vi "GOLPI Package Assistant Panel.vi"(8 "error in":errorcluster, 11 "golpi ref":T1) -> (0 "error out":errorcluster)   [LabVIEW 2013]
doc: "GOLPI package assistant panel."
uses:
  golpi_session_ref.ctl
  golpi_session.ctl
  GOLPI Library.lvlibp/Public/GOLPI reference Type Def.ctl
  GOLPI Library.lvlibp/LV Process source distribution/Pipe Handle.ctl
  GOLPI Library.lvlibp/Private/Get Variable - polymorph parts/Get Double.vi
  <vilib>/regexp/Match Regular Expression.xnode
  GOLPI Multi Process.lvlib
  GOLPI Library.lvlibp
  varilib/varilib.lvlib
  GOLPI Library.lvlibp/LV Process source distribution/LV Process library.lvlib
panel:
  in  "btn install":bool
  in  "btn clr":bool
  in  "btn rem":bool
  in  "btn add":bool
  in  "btn reload":bool
  in  "pkg select":i32(listbox) caption="Packages to load"
  in  "pkg list":i32(listbox) caption="Installed packages"
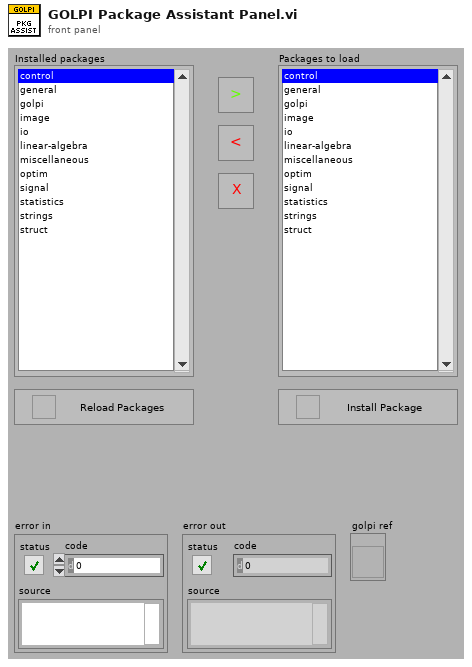
[diagram p1: front panel]
types:
  T1 = typedef "GOLPI Multi Process.lvlib/golpi_session_ref.ctl" = refnum<vi>
  T2 = typedef "GOLPI Package Assistant Actions" = enum16{"Reload packages"}
  T3 = typedef "GOLPI Library.lvlibp/GOLPI reference Type Def.ctl" = cluster{"pipe handle":T4, "fast read timeout [ms]":u32, "fast read settle time [ms]":u32, "fast read to multiple [ms]":u32, "max elements per input line":u32, "slow read timeout [ms]":u32, "stdin double format specifier":string, "max elements per stdout output column":u32, "console mode bitstream":bool, "bitstream first read timeout [ms]":u32, "bitstream read timeout [ms]":u32, "struct transfer possible":bool, "matlab mode":bool}
  T4 = typedef "GOLPI Library.lvlibp/LV Process library.lvlib/Pipe Handle.ctl" = cluster{"lv_proc.dll file path":path, "process instance handle":u32[], "debug mode":bool, "debug data":cluster{"time":timestamp, "stdin":bool, "data":string}[]}
  T5 = typedef "GOLPI Multi Process.lvlib/golpi_session.ctl" = cluster{"GOLPI ref":T3, "idn str":string, "octave path":path, "work path":path, "start timeout [ms]":u32, "clr cache":bool, "console":bool, "binary":bool, "semaphore":T6, "initial command":string, "exit command":string, "matlab":bool, "pkg list":string[]}
  T6 = typedef "Semaphore RefNum" = refnum<k1>
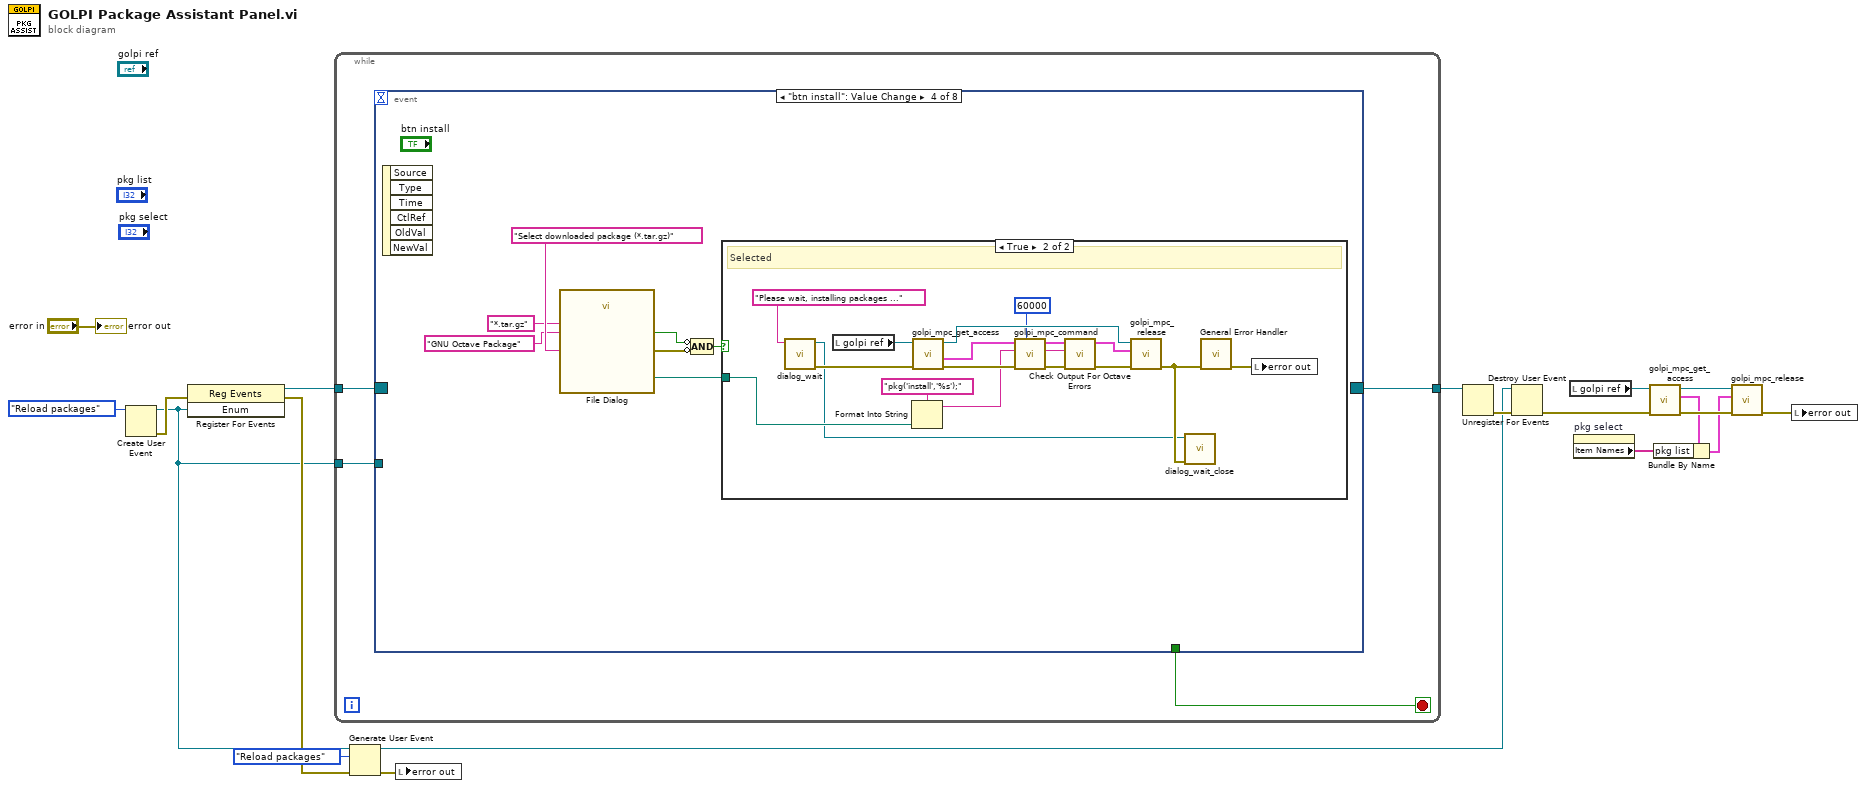
[diagram p0: block diagram]
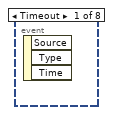
[diagram p2: hidden frame]
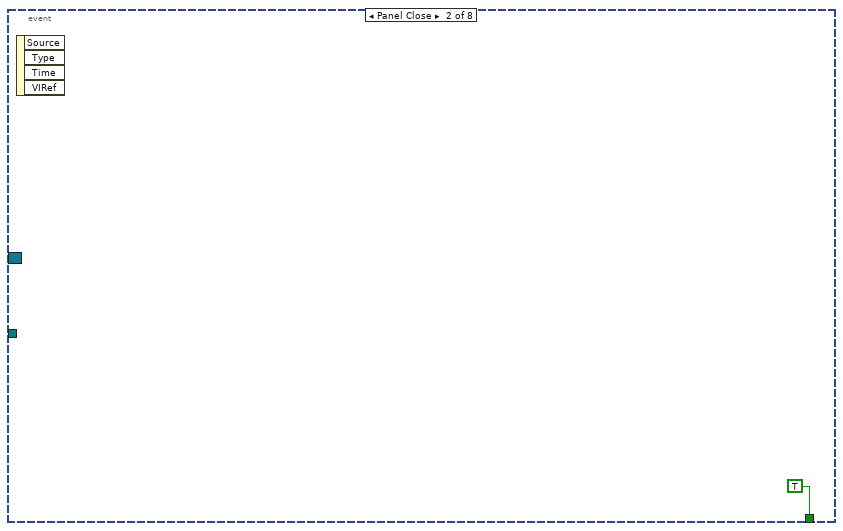
[diagram p3: hidden frame]
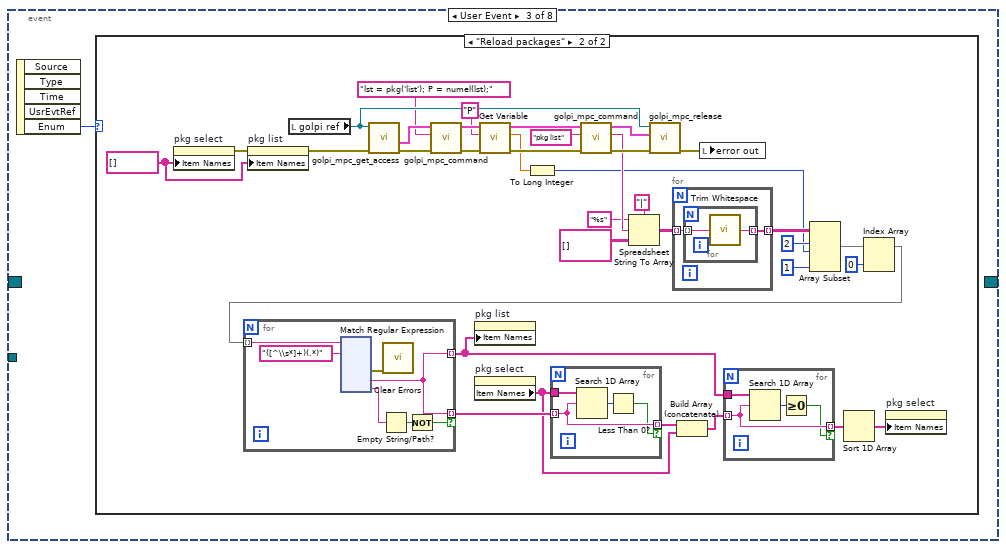
[diagram p4: hidden frame]
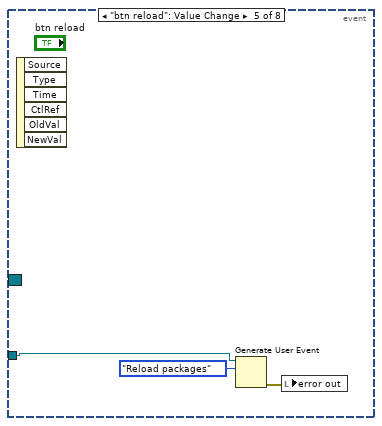
[diagram p7: hidden frame]
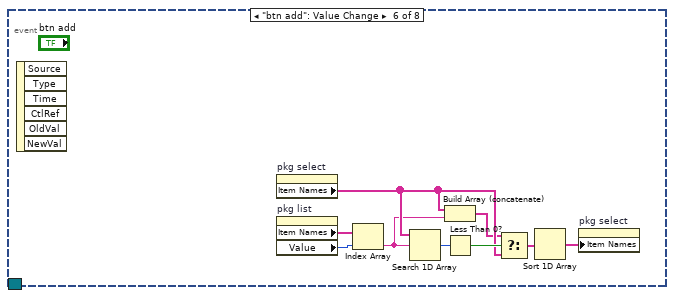
[diagram p8: hidden frame]
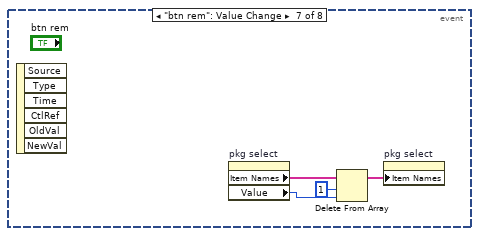
[diagram p9: hidden frame]
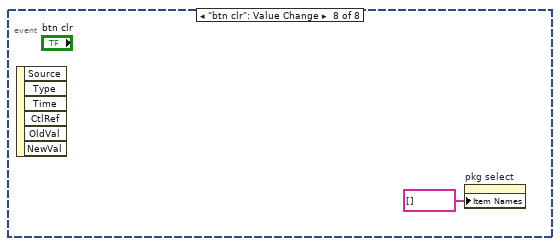
[diagram p10: hidden frame]
diagram:
  n1 = Create User Event(user event datatype=GOLPI_Package_Assistant_Actions."Reload packages" ("Enum")) -> (user event=w9:refnum<user-event>, error out=w14:errorcluster)  [unwired: 1 in]
  n2 = register-events(error in=w14, w9) -> (reference out=w17:refnum<event-registration>, error out=w12:errorcluster)  [unwired: 1 in]
  n3 = while {
    tunnel: w17 -> [w22]
    tunnel: [w21] -> w16
    tunnel: w9 -> [w20]
    stop <- w23 stop-if-true
    n4 = event shown="[3] \"btn install\": Value Change" {
      selector: w22 -> [_ _ _ _ _ _ _ _]
      dyn-events: [_ _ _ _ _ _ _ _] -> w21
      timeout: _ -> [_ _ _ _ _ _ _ _]
      tunnel: [_ TRUE _ _ _ _ _ _] -> w23
      tunnel: w20 -> [_ _ _ _ w223 _ _ _]
      event Timeout {
        n5 = event-data() -> ()  [unwired: 1 in, 3 out]
      }
      event Panel Close {
        n6 = event-data() -> ()  [unwired: 1 in, 4 out]
      }
      event User Event {
        n7 = event-data() -> ("Enum"=w25:T2)  [unwired: 1 in, 4 out]
        n8 = case shown="\"Reload packages\"" w25 {
          frame Default {
          }
          frame "Reload packages" {
            w26 = string[] [] ("Item Names")
            n9 = property on="pkg select" class="LstBox (strict)"("Item Names"=w26) -> (error out=w27:errorcluster)  [unwired: 2 in, 1 out]
            n10 = property on="pkg list" class="LstBox (strict)"(error in=w27, "Item Names"=w26) -> (error out=w28:errorcluster)  [unwired: 1 in, 1 out]
            n11 = local read "golpi ref"() -> (w58:T1)
            n12 = call "golpi_mpc_get_access.vi"("error in"=w28, "golpi session ref"=w58) -> ("error out"=w48:errorcluster, "GOLPI ref out"=w47:T3)  [unwired: 4 in, 4 out]
            n13 = call "golpi_mpc_command.vi"("error in"=w48, "command"="lst = pkg('list'); P = numel(lst);", "GOLPI ref in"=w47) -> ("error out"=w45:errorcluster, "GOLPI ref. out"=w44:T3)  [unwired: 6 in, 1 out]
            n14 = property on="pkg select" class="LstBox (strict)"() -> ("Item Names"=w33:string[])  [unwired: 2 in, 2 out]
            n15 = call-poly "Get Variable.vi"("error in"=w45, "variable name"="P", "GOLPI ref. in"=w44) -> ("error out"=w42:errorcluster, "value"=w40:dbl, "GOLPI ref. out"=w41:T3)  [unwired: 6 in]
            n16 = To Long Integer(number=w40) -> (32bit integer=w39:i32)
            n17 = call "golpi_mpc_command.vi"("error in"=w42, "command"="pkg list", "GOLPI ref in"=w41) -> ("error out"=w60:errorcluster, "read buffer"=w55:string, "GOLPI ref. out"=w59:T3)  [unwired: 6 in]
            n18 = Spreadsheet String To Array(delimiter (Tab)="|", format string="%s", spreadsheet string=w55, array type (2D Dbl)=string[][] []) -> (array=w52:string[][])
            n19 = call "golpi_mpc_release.vi"("error in"=w60, "golpi ref or golpi session in"=w59, "golpi session ref"=w58) -> ("error out"=w57:errorcluster)  [unwired: 7 in, 1 out]
            n20 = for {
              tunnel: w52 -> [w195] mode=indexing
              tunnel: [w194] -> w51 mode=indexing
              n21 = for {
                tunnel: w195 -> [w197] mode=indexing
                tunnel: [w196] -> w194 mode=indexing
                n22 = call <vilib>:"Trim Whitespace.vi"("string"=w197) -> ("trimmed string"=w196:string)  [unwired: 1 in]
              }
            }
            n23 = local write "error out"(w57) -> ()
            n24 = Array Subset(array=w51, index (row)=2 ("index"), length (row)=w39, length (col)=1 ("length")) -> (w38:string[][])  [unwired: 1 in]
            n25 = Index Array(array=w38, index (col)=0 ("disabled index (col)")) -> (element=w37:string[])  [unwired: 1 in]
            n26 = for {
              tunnel: w37 -> [w76] mode=indexing
              tunnel: [w72] -> w32 mode=indexing
              tunnel: [w72] -> w34 mode=indexing if=w70
              n27 = xnode "Match Regular Expression"("input string"=w76, "regular expression"="([^\\s*]+)(.*)") -> ("error out"=w75:errorcluster, "submatch 1"=w72:string, "submatch 2"=w73:string)  [unwired: 4 in, 4 out]
              n28 = Empty String/Path?(string/path=w73) -> (empty?=w71:bool)
              n29 = call <vilib>:"Clear Errors.vi"("error in (no error)"=w75) -> ()  [unwired: 6 in, 1 out]
              n30 = Not(x=w71) -> (.not. x?=w70:bool)
            }
            n31 = property on="pkg list" class="LstBox (strict)"("Item Names"=w32) -> ()  [unwired: 2 in, 2 out]
            n32 = for {
              tunnel: w34 -> [w67] mode=indexing
              tunnel: w33 -> [w69]
              tunnel: [w67] -> w35 mode=indexing if=w66
              n33 = Search 1D Array(1D array=w69, element=w67) -> (index of element=w68:i32)  [unwired: 1 in]
              n34 = Less Than 0?(x=w68) -> (x < 0?=w66:bool)
            }
            n35 = Build Array (concatenate)(w35, w33) -> (w31:string[])
            n36 = for {
              tunnel: w31 -> [w63] mode=indexing
              tunnel: w32 -> [w65]
              tunnel: [w63] -> w30 mode=indexing if=w62
              n37 = Search 1D Array(1D array=w65, element=w63) -> (index of element=w64:i32)  [unwired: 1 in]
              n38 = Greater Or Equal To 0?(x=w64) -> (x >= 0?=w62:bool)
            }
            n39 = Sort 1D Array(array=w30) -> (sorted array=w29:string[])
            n40 = property on="pkg select" class="LstBox (strict)"("Item Names"=w29) -> ()  [unwired: 2 in, 2 out]
          }
        }
      }
      event "btn install": Value Change {
        n41 = event-data() -> ()  [unwired: 1 in, 6 out]
        n42 = call "File Dialog"("prompt"="Select downloaded package (*.tar.gz)", "pattern (all files)"="*.tar.gz", "pattern label"="GNU Octave Package") -> ("selected path"=w198:path, "cancelled"=w200:bool, "error out"=w201:errorcluster)  [unwired: 9 in, 1 out]
        n43 = Compound Arithmetic op=AND(invert w200, invert w201) -> (w199:bool)
        n44 = case shown="True" w199 {
          tunnel: w198 -> [_ w212]
          frame False {
          }
          frame True {
            # "Selected"
            n45 = call "dialog_wait.vi"("message string"="Please wait, installing packages ...") -> ("error out"=w208:errorcluster, "reference out"=w205:refnum<vi>)  [unwired: 9 in]
            n46 = local read "golpi ref"() -> (w221:T1)
            n47 = Format Into String(format string="pkg('install','%s');", w212) -> (resulting string=w210:string)  [unwired: 2 in, 1 out]
            n48 = call "golpi_mpc_get_access.vi"("error in"=w208, "golpi session ref"=w221) -> ("error out"=w219:errorcluster, "GOLPI ref out"=w214:T3, "golpi session ref out (copy)"=w220:T1)  [unwired: 4 in, 3 out]
            n49 = call "golpi_mpc_command.vi"("timeout [ms]"=u32 60000, "error in"=w219, "command"=w210, "GOLPI ref in"=w214) -> ("error out"=w217:errorcluster, "read buffer"=w216:string, "GOLPI ref. out"=w213:T3)  [unwired: 5 in]
            n50 = call "Check Output For Octave Errors.vi"("error in"=w217, "read buffer"=w216) -> ("error out"=w215:errorcluster)  [unwired: 9 in]
            n51 = call "golpi_mpc_release.vi"("error in"=w215, "golpi ref or golpi session in"=w213, "golpi session ref"=w220) -> ("error out"=w206:errorcluster)  [unwired: 7 in, 1 out]
            n52 = call "dialog_wait_close.vi"("error in"=w206, "async vi ref"=w205) -> ()  [unwired: 2 in]
            n53 = call <vilib>:"General Error Handler.vi"("error in (no error)"=w206) -> ("error out"=w209:errorcluster)  [unwired: 10 in, 4 out]
            n54 = local write "error out"(w209) -> ()
          }
        }
      }
      event "btn reload": Value Change {
        n55 = event-data() -> ()  [unwired: 1 in, 6 out]
        n56 = Generate User Event(user event=w223, event data cluster=GOLPI_Package_Assistant_Actions."Reload packages" ("event data")) -> (error out=w224:errorcluster)  [unwired: 2 in, 1 out]
        n57 = local write "error out"(w224) -> ()
      }
      event "btn add": Value Change {
        n58 = event-data() -> ()  [unwired: 1 in, 6 out]
        n59 = property on="pkg select" class="LstBox (strict)"() -> ("Item Names"=w229:string[])  [unwired: 2 in, 2 out]
        n60 = property on="pkg list" class="LstBox (strict)"() -> ("Item Names"=w233:string[], "Value"=w232:i32)  [unwired: 2 in, 2 out]
        n61 = Index Array(array=w233, index=w232) -> (element=w228:string)
        n62 = Search 1D Array(1D array=w229, element=w228) -> (index of element=w231:i32)  [unwired: 1 in]
        n63 = Build Array (concatenate)(w229, w228) -> (w227:string[])
        n64 = Less Than 0?(x=w231) -> (x < 0?=w230:bool)
        n65 = Select(t=w227, s=w230, f=w229) -> (s? t:f=w226:string[])
        n66 = Sort 1D Array(array=w226) -> (sorted array=w225:string[])
        n67 = property on="pkg select" class="LstBox (strict)"("Item Names"=w225) -> ()  [unwired: 2 in, 2 out]
      }
      event "btn rem": Value Change {
        n68 = event-data() -> ()  [unwired: 1 in, 6 out]
        n69 = property on="pkg select" class="LstBox (strict)"() -> ("Item Names"=w237:string[], "Value"=w236:i32)  [unwired: 2 in, 2 out]
        n70 = Delete From Array(array=w237, length=1, index=w236) -> (array with subset deleted=w234:string[])  [unwired: 1 out]
        n71 = property on="pkg select" class="LstBox (strict)"("Item Names"=w234) -> ()  [unwired: 2 in, 2 out]
      }
      event "btn clr": Value Change {
        n72 = event-data() -> ()  [unwired: 1 in, 6 out]
        n73 = property on="pkg select" class="LstBox (strict)"("Item Names"=string[] []) -> ()  [unwired: 2 in, 2 out]
      }
    }
  }
  n74 = Generate User Event(user event=w9, event data cluster=GOLPI_Package_Assistant_Actions."Reload packages" ("event data"), error in=w12) -> (user event out=w13:refnum<user-event>, error out=w11:errorcluster)  [unwired: 1 in]
  n75 = local write "error out"(w11) -> ()
  n76 = Unregister For Events(event registration refnum=w16) -> (error out=w15:errorcluster)  [unwired: 1 in]
  n77 = Destroy User Event(user event=w13, error in=w15) -> (error out=w2:errorcluster)
  n78 = local read "golpi ref"() -> (w8:T1)
  n79 = property on="pkg select" class="LstBox (strict)"() -> ("Item Names"=w3:string[])  [unwired: 2 in, 2 out]
  n80 = call "golpi_mpc_get_access.vi"("error in"=w2, "golpi session ref"=w8) -> ("error out"=w7:errorcluster, "golpi session out"=w6:T5, "golpi session ref out (copy)"=w4:T1)  [unwired: 4 in, 3 out]
  n81 = Bundle By Name(cluster=w6, "pkg list"=w3) -> (w5:T5)
  n82 = call "golpi_mpc_release.vi"("error in"=w7, "golpi ref or golpi session in"=w5, "golpi session ref"=w4) -> ("error out"=w1:errorcluster)  [unwired: 7 in, 1 out]
  n83 = local write "error out"(w1) -> ()
  "error out" <- "error in"
